vi "Central.vi"() -> ()   [LabVIEW 2017]
uses:
  Desktop/New folder (2)/Selectable ListBox xControl/ListBox XControl.xctl
panel:
  in  "?":bool
  in  "End":timestamp format="%<%.3X>T"
  in  "Start":timestamp format="%<%.3X>T"
  in  "Get":bool
  in  "TimeSlot Name":string
  out "Selected Items []":string[](array[string])
  out "Selected Index []":i32[](array[numeric])
  in  "ListBox XControl":string[](xcontrol)
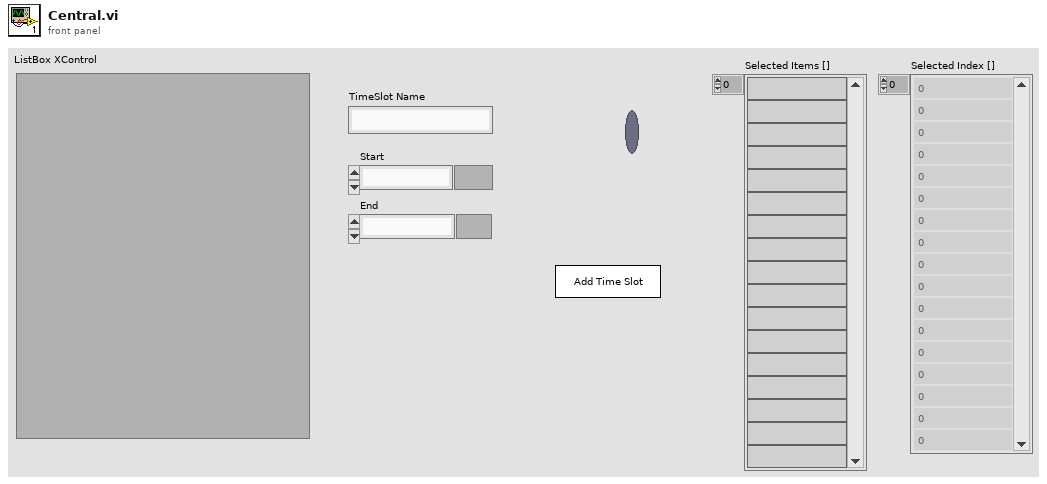
[diagram p1: front panel]
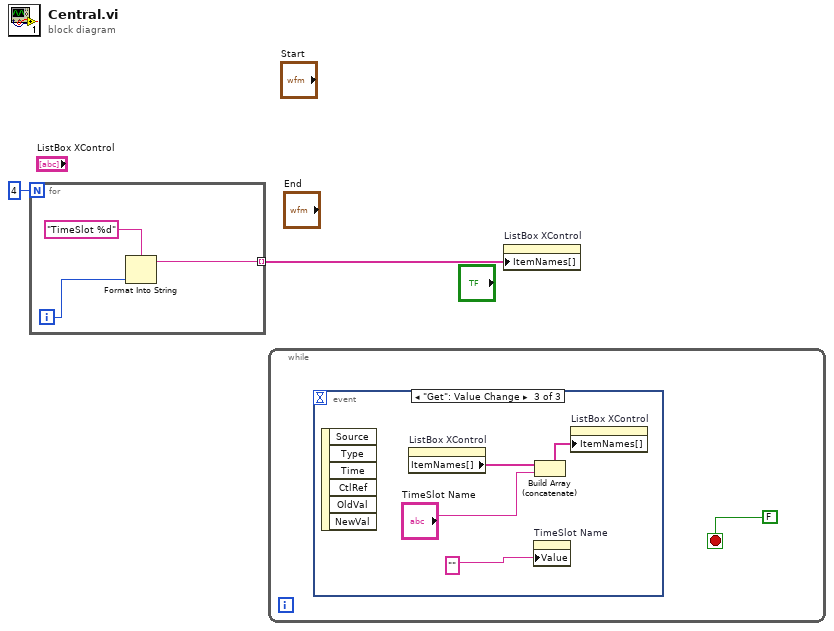
[diagram p0: block diagram]
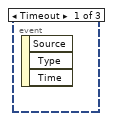
[diagram p2: hidden frame]
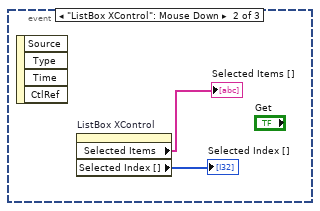
[diagram p3: hidden frame]
diagram:
  n1 = for {
    N: 4 -> [_]
    tunnel: [w3] -> w2 mode=indexing
    i -> [w5]
    n2 = Format Into String(format string="TimeSlot %d", w5) -> (resulting string=w3:string)  [unwired: 2 in, 1 out]
  }
  n3 = while {
    stop <- FALSE stop-if-true
    n4 = event shown="[2] \"Get\": Value Change" {
      selector: _ -> [_ _ _]
      dyn-events: _ -> [_ _ _]
      timeout: _ -> [_ _ _]
      event Timeout {
        n5 = event-data() -> ()  [unwired: 1 in, 3 out]
      }
      event "ListBox XControl": Mouse Down {
        n6 = event-data() -> ()  [unwired: 1 in, 4 out]
        n7 = property on="ListBox XControl" class="ListBox XControl (strict)"() -> ("Selected Items"=→"Selected Items []":string[], "Selected Index []"=→"Selected Index []":i32[])  [unwired: 2 in, 2 out]
      }
      event "Get": Value Change {
        n8 = event-data() -> ()  [unwired: 1 in, 6 out]
        n9 = property on="ListBox XControl" class="ListBox XControl (strict)"() -> ("ItemNames[]"=w12:string[])  [unwired: 2 in, 2 out]
        n10 = property on="TimeSlot Name" class="Str"("Value"="") -> ()  [unwired: 2 in, 2 out]
        n11 = Build Array (concatenate)(w12, "TimeSlot Name") -> (w9:string[])
        n12 = property on="ListBox XControl" class="ListBox XControl (strict)"("ItemNames[]"=w9) -> ()  [unwired: 2 in, 2 out]
      }
    }
  }
  n13 = property on="ListBox XControl" class="ListBox XControl (strict)"("ItemNames[]"=w2) -> ()  [unwired: 2 in, 2 out]
